vi "Next Page.vi"(8 "error in (no error)":errorcluster, 11 "Test Channel Model in":refnum<class "Test Channel Model.lvclass">) -> (0 "error out":errorcluster, 3 "Test Channel Model out":refnum<class "Test Channel Model.lvclass">)   [LabVIEW 2013, in "Test Channel Model.lvlib" / "Test Channel Model.lvclass"]
uses:
  Test Channel Model.lvclass
  Test Channel Model.lvclass/Test Channel Model.ctl
  <vilib>/ActorFrameworkMVC/View Observer/View Registry/View Registry.lvclass/View Registry.ctl
  Test Channel Model Messages/Abstract Test Channel Move In Next Msg/Abstract Test Channel Move In Next Msg.lvclass
  <vilib>/ActorFrameworkMVC/View Observer/View Registry/View Registry.lvclass
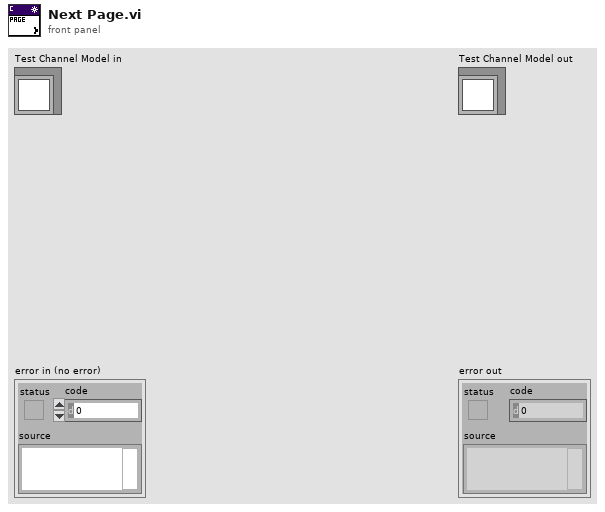
[diagram p1: front panel]
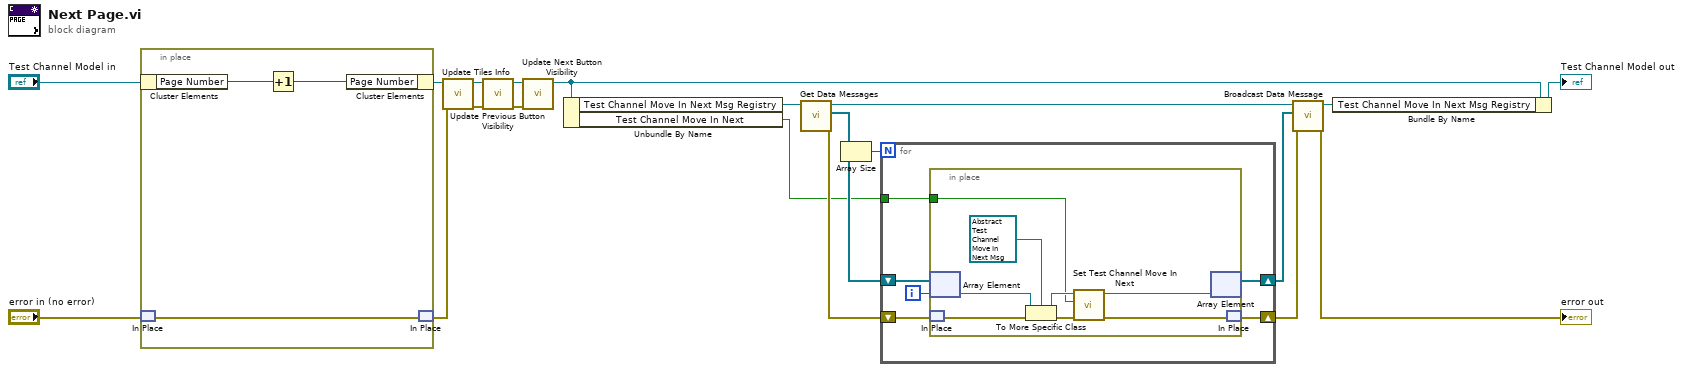
[diagram p0: block diagram]
diagram:
  n1 = in-place {
    n2 = in-place-cluster #1("Test Channel Model in") -> ("Page Number"=w23:i32)
    n3 = in-place-match #2("error in (no error)") -> (w21:errorcluster)
    n4 = Increment(x=w23) -> (x+1=w22:i32)
    n5 = in-place-cluster #1("Page Number"=w22) -> (w13:refnum<class "Test Channel Model.lvclass">)
    n6 = in-place-match #2(w21) -> (w8:errorcluster)
  }
  n7 = call "Update Tiles Info.vi"("error in (no error)"=w8, "Test Channel Model in"=w13) -> ("error out"=w7:errorcluster, "Test Channel Model out"=w12:refnum<class "Test Channel Model.lvclass">)  [unwired: 8 in]
  n8 = call "Update Previous Button Visibility.vi"("error in (no error)"=w7, "Test Channel Model in"=w12) -> ("error out"=w6:errorcluster, "Test Channel Model out"=w11:refnum<class "Test Channel Model.lvclass">)  [unwired: 8 in]
  n9 = call "Update Next Button Visibility.vi"("error in (no error)"=w6, "Test Channel Model in"=w11) -> ("Test Channel Model out"=w2:refnum<class "Test Channel Model.lvclass">)  [unwired: 8 in, 1 out]
  n10 = Unbundle By Name(w2) -> ("Test Channel Move In Next Msg Registry"=w10:refnum<class "View Registry.lvclass">, "Test Channel Move In Next"=w14:bool)
  n11 = call <vilib>:"Get Data Messages.vi"("View Registry in"=w10) -> ("error out"=w18:errorcluster, "Data Messages"=w19:refnum<class "Data Message.lvclass">[], "View Registry out"=w9:refnum<class "View Registry.lvclass">)  [unwired: 8 in]
  n12 = Array Size(array=w19) -> (size(s)=w20:i32)
  n13 = for {
    N: w20 -> [_]
    shift-right: [w28] -> w17
    shift-left: w19 -> [w29]
    shift-right: [w25] -> w16
    shift-left: w18 -> [w27]
    tunnel: w14 -> [w26]
    i -> [w24]
    n14 = in-place {
      in-place-border: w26 -> [w30]
      n15 = in-place-array #3(w29, w24) -> (w35:refnum<class "Data Message.lvclass">)
      n16 = in-place-match #4(w27) -> (w37:errorcluster)
      n17 = To More Specific Class(target class=refnum<class "Abstract Test Channel Move In Next Msg.lvclass"> refnum ("Test Channel Model.lvlib:Abstract Test Channel Move In Next Msg.lvclass"), reference=w35, error in=w37) -> (specific class reference=w31:refnum<class "Abstract Test Channel Move In Next Msg.lvclass">, error out=w34:errorcluster)
      n18 = call "Set Test Channel Move In Next.vi"("error in (no error)"=w34, "Test Channel Move In Next"=w30, "Abstract Test Channel Move In Next Msg in"=w31) -> ("error out"=w33:errorcluster, "Abstract Test Channel Move In Next Msg out"=w32:refnum<class "Abstract Test Channel Move In Next Msg.lvclass">)  [unwired: 7 in]
      n19 = in-place-array #3(w32) -> (w28:refnum<class "Data Message.lvclass">[])  [unwired: 1 out]
      n20 = in-place-match #4(w33) -> (w25:errorcluster)
    }
  }
  n21 = call <vilib>:"Broadcast Data Message.vi"("error in (no error)"=w16, "Data Messages"=w17, "View Registry in"=w9) -> ("error out"=→"error out":errorcluster, "View Registry out"=w15:refnum<class "View Registry.lvclass">)  [unwired: 7 in]
  n22 = Bundle By Name(cluster=w2, "Test Channel Move In Next Msg Registry"=w15) -> (→"Test Channel Model out":refnum<class "Test Channel Model.lvclass">)
